vi "Package from File.vi"(8 "error in (no error)":errorcluster, 10 "GPack File":refnum<class "GPack File.lvclass">) -> (0 "error out":errorcluster, 2 "PackageAbstract":refnum<class "PackageAbstract.lvclass">)   [LabVIEW 2020, in "GPack.lvlib"]
uses:
  GPack.lvlib
  GPack File/GPack File.lvclass
  PackageAbstract/PackageAbstract.lvclass
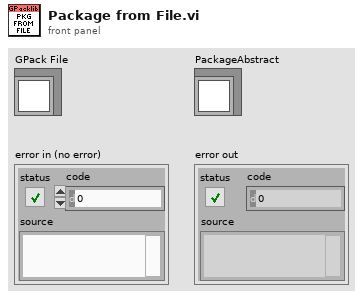
[diagram p1: front panel]
types:
  T1 = typedef "GPack.lvlib/Package Info.ctl" = cluster{"Name":string, "Type":string, "Host":string, "Path":string, "Branch":string, "Version":string}
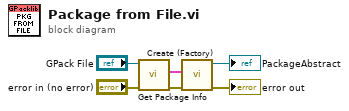
[diagram p0: block diagram]
diagram:
  n1 = call "Get Package Info.vi"("GPack File in"="GPack File") -> ("Package Info"=w3:T1)  [unwired: 10 in]
  n2 = call "Create (Factory).vi"("error in (no error)"="error in (no error)", "Package Info"=w3) -> ("error out"=→"error out":errorcluster, "PackageAbstract out"=→"PackageAbstract":refnum<class "PackageAbstract.lvclass">)  [unwired: 8 in]
